vi "Modbus Master全局变量.vi"() -> ()   [LabVIEW 2016, in "数据传输系统-02.lvlib"]
panel:
  out "数组":dbl[](array[numeric])
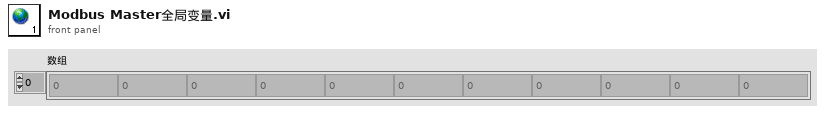
[diagram p1: front panel]
diagram:
